vi "rsidr_core_global.vi"() -> ()   [LabVIEW 2015, in "Rohde&Schwarz CMXP NR FR2 Measurement.lvlib"] (continued)
"Access"=enum."Read Only", "Range Table"="", "Read Callback"="", "Write Callback"="", "Range Callback"="", "Check Callback"="", "Rngtable Callback"="", "Coerce Callback"="", "Supported Models"="", "Instrument Options"="", "Check Status Callback"="", "Flags"=0, "Help"="Returns equalizer spectrum flatness single value results (maximum within a range) for all measured list mode segments.\n\nAvailable Repeated Capabilities:\ninstance: i0, i1, i2, i3, i4, i5, i6, i7, i8, i9, i10, i11, i12, i13, i14, i15, i16, i17, i18, i19, i20, i21, i22, i23, i24, i25, i26, i27, i28, i29, i30, i31, i32\r\nRange: r1, r2\r\n\nRemote-control command(s):\nFETCh:NRMMw:MEAS<i>:MEValuation:LIST:ESFLatness:MAXR<no>:CURRent?"}, {"Level"=5, "Class Only"=FALSE, "Identifier"="RSCMXPNRFR2M_ATTR_FETCH_MULTI_EVAL_MEASUREMENT_LIST_ESF_MAXR_EXTREME_RESULTS", "Descriptive Name"="Fetch Multi Eval Measurement List ES Flatness MaxR Extreme Results", "Data Type"=enum."RawString", "Command"="FETC:NRMM:MEAS{instance}:MEV:LIST:ESFL:MAXR{Range}:EXTR?", "Access"=enum."Read Only", "Range Table"="", "Read Callback"="", "Write Callback"="", "Range Callback"="", "Check Callback"="", "Rngtable Callback"="", "Coerce Callback"="", "Supported Models"="", "Instrument Options"="", "Check Status Callback"="", "Flags"=0, "Help"="Returns equalizer spectrum flatness single value results (maximum within a range) for all measured list mode segments.\n\nAvailable Repeated Capabilities:\ninstance: i0, i1, i2, i3, i4, i5, i6, i7, i8, i9, i10, i11, i12, i13, i14, i15, i16, i17, i18, i19, i20, i21, i22, i23, i24, i25, i26, i27, i28, i29, i30, i31, i32\r\nRange: r1, r2\r\n\nRemote-control command(s):\nFETCh:NRMMw:MEAS<i>:MEValuation:LIST:ESFLatness:MAXR<no>:EXTReme?"}, {"Level"=5, "Class Only"=FALSE, "Identifier"="RSCMXPNRFR2M_ATTR_FETCH_MULTI_EVAL_MEASUREMENT_LIST_ESF_MAXR_STANDARD_DEVIATION_RESULTS", "Descriptive Name"="Fetch Multi Eval Measurement List ES Flatness MaxR Standard Deviation Results", "Data Type"=enum."RawString", "Command"="FETC:NRMM:MEAS{instance}:MEV:LIST:ESFL:MAXR{Range}:SDEV?", "Access"=enum."Read Only", "Range Table"="", "Read Callback"="", "Write Callback"="", "Range Callback"="", "Check Callback"="", "Rngtable Callback"="", "Coerce Callback"="", "Supported Models"="", "Instrument Options"="", "Check Status Callback"="", "Flags"=0, "Help"="Returns equalizer spectrum flatness single value results (maximum within a range) for all measured list mode segments.\n\nAvailable Repeated Capabilities:\ninstance: i0, i1, i2, i3, i4, i5, i6, i7, i8, i9, i10, i11, i12, i13, i14, i15, i16, i17, i18, i19, i20, i21, i22, i23, i24, i25, i26, i27, i28, i29, i30, i31, i32\r\nRange: r1, r2\r\n\nRemote-control command(s):\nFETCh:NRMMw:MEAS<i>:MEValuation:LIST:ESFLatness:MAXR<no>:SDEViation?"}, {"Level"=5, "Class Only"=FALSE, "Identifier"="RSCMXPNRFR2M_ATTR_QUERY_MULTI_EVAL_MEASUREMENT_LIST_ESF_MAXR_AVERAGE_LIMIT_CHECK_RESULTS", "Descriptive Name"="Query Multi Eval Measurement List ES Flatness MaxR Average Limit Check Results", "Data Type"=enum."RawString", "Command"="CALC:NRMM:MEAS{instance}:MEV:LIST:ESFL:MAXR{Range}:AVER?", "Access"=enum."Read Only", "Range Table"="", "Read Callback"="", "Write Callback"="", "Range Callback"="", "Check Callback"="", "Rngtable Callback"="", "Coerce Callback"="", "Supported Models"="", "Instrument Options"="", "Check Status Callback"="", "Flags"=0, "Help"="Returns the limit check results for equalizer spectrum flatness single value results (maximum within a range) for all measured list mode segments.\n\nAvailable Repeated Capabilities:\ninstance: i0, i1, i2, i3, i4, i5, i6, i7, i8, i9, i10, i11, i12, i13, i14, i15, i16, i17, i18, i19, i20, i21, i22, i23, i24, i25, i26, i27, i28, i29, i30, i31, i32\r\nRange: r1, r2\r\n\nRemote-control command(s):\nCALCulate:NRMMw:MEAS<i>:MEValuation:LIST:ESFLatness:MAXR<no>:AVERage?"}, {"Level"=5, "Class Only"=FALSE, "Identifier"="RSCMXPNRFR2M_ATTR_QUERY_MULTI_EVAL_MEASUREMENT_LIST_ESF_MAXR_CURRENT_LIMIT_CHECK_RESULTS", "Descriptive Name"="Query Multi Eval Measurement List ES Flatness MaxR Current Limit Check Results", "Data Type"=enum."RawString", "Command"="CALC:NRMM:MEAS{instance}:MEV:LIST:ESFL:MAXR{Range}:CURR?", "Access"=enum."Read Only", "Range Table"="", "Read Callback"="", "Write Callback"="", "Range Callback"="", "Check Callback"="", "Rngtable Callback"="", "Coerce Callback"="", "Supported Models"="", "Instrument Options"="", "Check Status Callback"="", "Flags"=0, "Help"="Returns the limit check results for equalizer spectrum flatness single value results (maximum within a range) for all measured list mode segments.\n\nAvailable Repeated Capabilities:\ninstance: i0, i1, i2, i3, i4, i5, i6, i7, i8, i9, i10, i11, i12, i13, i14, i15, i16, i17, i18, i19, i20, i21, i22, i23, i24, i25, i26, i27, i28, i29, i30, i31, i32\r\nRange: r1, r2\r\n\nRemote-control command(s):\nCALCulate:NRMMw:MEAS<i>:MEValuation:LIST:ESFLatness:MAXR<no>:CURRent?"}, {"Level"=5, "Class Only"=FALSE, "Identifier"="RSCMXPNRFR2M_ATTR_QUERY_MULTI_EVAL_MEASUREMENT_LIST_ESF_MAXR_EXTREME_LIMIT_CHECK_RESULTS", "Descriptive Name"="Query Multi Eval Measurement List ES Flatness MaxR Extreme Limit Check Results", "Data Type"=enum."RawString", "Command"="CALC:NRMM:MEAS{instance}:MEV:LIST:ESFL:MAXR{Range}:EXTR?", "Access"=enum."Read Only", "Range Table"="", "Read Callback"="", "Write Callback"="", "Range Callback"="", "Check Callback"="", "Rngtable Callback"="", "Coerce Callback"="", "Supported Models"="", "Instrument Options"="", "Check Status Callback"="", "Flags"=0, "Help"="Returns the limit check results for equalizer spectrum flatness single value results (maximum within a range) for all measured list mode segments.\n\nAvailable Repeated Capabilities:\ninstance: i0, i1, i2, i3, i4, i5, i6, i7, i8, i9, i10, i11, i12, i13, i14, i15, i16, i17, i18, i19, i20, i21, i22, i23, i24, i25, i26, i27, i28, i29, i30, i31, i32\r\nRange: r1, r2\r\n\nRemote-control command(s):\nCALCulate:NRMMw:MEAS<i>:MEValuation:LIST:ESFLatness:MAXR<no>:EXTReme?"}, {"Level"=5, "Class Only"=FALSE, "Identifier"="RSCMXPNRFR2M_ATTR_FETCH_MULTI_EVAL_MEASUREMENT_LIST_ESF_MINR_AVERAGE_RESULTS", "Descriptive Name"="Fetch Multi Eval Measurement List ES Flatness MinR Average Results", "Data Type"=enum."RawString", "Command"="FETC:NRMM:MEAS{instance}:MEV:LIST:ESFL:MINR{Range}:AVER?", "Access"=enum."Read Only", "Range Table"="", "Read Callback"="", "Write Callback"="", "Range Callback"="", "Check Callback"="", "Rngtable Callback"="", "Coerce Callback"="", "Supported Models"="", "Instrument Options"="", "Check Status Callback"="", "Flags"=0, "Help"="Returns equalizer spectrum flatness single value results (minimum within a range) for all measured list mode segments.\n\nAvailable Repeated Capabilities:\ninstance: i0, i1, i2, i3, i4, i5, i6, i7, i8, i9, i10, i11, i12, i13, i14, i15, i16, i17, i18, i19, i20, i21, i22, i23, i24, i25, i26, i27, i28, i29, i30, i31, i32\r\nRange: r1, r2\r\n\nRemote-control command(s):\nFETCh:NRMMw:MEAS<i>:MEValuation:LIST:ESFLatness:MINR<no>:AVERage?"}, {"Level"=5, "Class Only"=FALSE, "Identifier"="RSCMXPNRFR2M_ATTR_FETCH_MULTI_EVAL_MEASUREMENT_LIST_ESF_MINR_CURRENT_RESULTS", "Descriptive Name"="Fetch Multi Eval Measurement List ES Flatness MinR Current Results", "Data Type"=enum."RawString", "Command"="FETC:NRMM:MEAS{instance}:MEV:LIST:ESFL:MINR{Range}:CURR?", "Access"=enum."Read Only", "Range Table"="", "Read Callback"="", "Write Callback"="", "Range Callback"="", "Check Callback"="", "Rngtable Callback"="", "Coerce Callback"="", "Supported Models"="", "Instrument Options"="", "Check Status Callback"="", "Flags"=0, "Help"="Returns equalizer spectrum flatness single value results (minimum within a range) for all measured list mode segments.\n\nAvailable Repeated Capabilities:\ninstance: i0, i1, i2, i3, i4, i5, i6, i7, i8, i9, i10, i11, i12, i13, i14, i15, i16, i17, i18, i19, i20, i21, i22, i23, i24, i25, i26, i27, i28, i29, i30, i31, i32\r\nRange: r1, r2\r\n\nRemote-control command(s):\nFETCh:NRMMw:MEAS<i>:MEValuation:LIST:ESFLatness:MINR<no>:CURRent?"}, {"Level"=5, "Class Only"=FALSE, "Identifier"="RSCMXPNRFR2M_ATTR_FETCH_MULTI_EVAL_MEASUREMENT_LIST_ESF_MINR_EXTREME_RESULTS", "Descriptive Name"="Fetch Multi Eval Measurement List ES Flatness MinR Extreme Results", "Data Type"=enum."RawString", "Command"="FETC:NRMM:MEAS{instance}:MEV:LIST:ESFL:MINR{Range}:EXTR?", "Access"=enum."Read Only", "Range Table"="", "Read Callback"="", "Write Callback"="", "Range Callback"="", "Check Callback"="", "Rngtable Callback"="", "Coerce Callback"="", "Supported Models"="", "Instrument Options"="", "Check Status Callback"="", "Flags"=0, "Help"="Returns equalizer spectrum flatness single value results (minimum within a range) for all measured list mode segments.\n\nAvailable Repeated Capabilities:\ninstance: i0, i1, i2, i3, i4, i5, i6, i7, i8, i9, i10, i11, i12, i13, i14, i15, i16, i17, i18, i19, i20, i21, i22, i23, i24, i25, i26, i27, i28, i29, i30, i31, i32\r\nRange: r1, r2\r\n\nRemote-control command(s):\nFETCh:NRMMw:MEAS<i>:MEValuation:LIST:ESFLatness:MINR<no>:EXTReme?"}, {"Level"=5, "Class Only"=FALSE, "Identifier"="RSCMXPNRFR2M_ATTR_FETCH_MULTI_EVAL_MEASUREMENT_LIST_ESF_MINR_STANDARD_DEVIATION_RESULTS", "Descriptive Name"="Fetch Multi Eval Measurement List ES Flatness MinR Standard Deviation Results", "Data Type"=enum."RawString", "Command"="FETC:NRMM:MEAS{instance}:MEV:LIST:ESFL:MINR{Range}:SDEV?", "Access"=enum."Read Only", "Range Table"="", "Read Callback"="", "Write Callback"="", "Range Callback"="", "Check Callback"="", "Rngtable Callback"="", "Coerce Callback"="", "Supported Models"="", "Instrument Options"="", "Check Status Callback"="", "Flags"=0, "Help"="Returns equalizer spectrum flatness single value results (minimum within a range) for all measured list mode segments.\n\nAvailable Repeated Capabilities:\ninstance: i0, i1, i2, i3, i4, i5, i6, i7, i8, i9, i10, i11, i12, i13, i14, i15, i16, i17, i18, i19, i20, i21, i22, i23, i24, i25, i26, i27, i28, i29, i30, i31, i32\r\nRange: r1, r2\r\n\nRemote-control command(s):\nFETCh:NRMMw:MEAS<i>:MEValuation:LIST:ESFLatness:MINR<no>:SDEViation?"}, {"Level"=5, "Class Only"=FALSE, "Identifier"="RSCMXPNRFR2M_ATTR_QUERY_MULTI_EVAL_MEASUREMENT_LIST_ESF_MINR_AVERAGE_LIMIT_CHECK_RESULTS", "Descriptive Name"="Query Multi Eval Measurement List ES Flatness MinR Average Limit Check Results", "Data Type"=enum."RawString", "Command"="CALC:NRMM:MEAS{instance}:MEV:LIST:ESFL:MINR{Range}:AVER?", "Access"=enum."Read Only", "Range Table"="", "Read Callback"="", "Write Callback"="", "Range Callback"="", "Check Callback"="", "Rngtable Callback"="", "Coerce Callback"="", "Supported Models"="", "Instrument Options"="", "Check Status Callback"="", "Flags"=0, "Help"="Returns the limit check results for equalizer spectrum flatness single value results (minimum within a range) for all measured list mode segments.\n\nAvailable Repeated Capabilities:\ninstance: i0, i1, i2, i3, i4, i5, i6, i7, i8, i9, i10, i11, i12, i13, i14, i15, i16, i17, i18, i19, i20, i21, i22, i23, i24, i25, i26, i27, i28, i29, i30, i31, i32\r\nRange: r1, r2\r\n\nRemote-control command(s):\nCALCulate:NRMMw:MEAS<i>:MEValuation:LIST:ESFLatness:MINR<no>:AVERage?"}, {"Level"=5, "Class Only"=FALSE, "Identifier"="RSCMXPNRFR2M_ATTR_QUERY_MULTI_EVAL_MEASUREMENT_LIST_ESF_MINR_CURRENT_LIMIT_CHECK_RESULTS", "Descriptive Name"="Query Multi Eval Measurement List ES Flatness MinR Current Limit Check Results", "Data Type"=enum."RawString", "Command"="CALC:NRMM:MEAS{instance}:MEV:LIST:ESFL:MINR{Range}:CURR?", "Access"=enum."Read Only", "Range Table"="", "Read Callback"="", "Write Callback"="", "Range Callback"="", "Check Callback"="", "Rngtable Callback"="", "Coerce Callback"="", "Supported Models"="", "Instrument Options"="", "Check Status Callback"="", "Flags"=0, "Help"="Returns the limit check results for equalizer spectrum flatness single value results (minimum within a range) for all measured list mode segments.\n\nAvailable Repeated Capabilities:\ninstance: i0, i1, i2, i3, i4, i5, i6, i7, i8, i9, i10, i11, i12, i13, i14, i15, i16, i17, i18, i19, i20, i21, i22, i23, i24, i25, i26, i27, i28, i29, i30, i31, i32\r\nRange: r1, r2\r\n\nRemote-control command(s):\nCALCulate:NRMMw:MEAS<i>:MEValuation:LIST:ESFLatness:MINR<no>:CURRent?"}, {"Level"=5, "Class Only"=FALSE, "Identifier"="RSCMXPNRFR2M_ATTR_QUERY_MULTI_EVAL_MEASUREMENT_LIST_ESF_MINR_EXTREME_LIMIT_CHECK_RESULTS", "Descriptive Name"="Query Multi Eval Measurement List ES Flatness MinR Extreme Limit Check Results", "Data Type"=enum."RawString", "Command"="CALC:NRMM:MEAS{instance}:MEV:LIST:ESFL:MINR{Range}:EXTR?", "Access"=enum."Read Only", "Range Table"="", "Read Callback"="", "Write Callback"="", "Range Callback"="", "Check Callback"="", "Rngtable Callback"="", "Coerce Callback"="", "Supported Models"="", "Instrument Options"="", "Check Status Callback"="", "Flags"=0, "Help"="Returns the limit check results for equalizer spectrum flatness single value results (minimum within a range) for all measured list mode segments.\n\nAvailable Repeated Capabilities:\ninstance: i0, i1, i2, i3, i4, i5, i6, i7, i8, i9, i10, i11, i12, i13, i14, i15, i16, i17, i18, i19, i20, i21, i22, i23, i24, i25, i26, i27, i28, i29, i30, i31, i32\r\nRange: r1, r2\r\n\nRemote-control command(s):\nCALCulate:NRMMw:MEAS<i>:MEValuation:LIST:ESFLatness:MINR<no>:EXTReme?"}, {"Level"=5, "Class Only"=FALSE, "Identifier"="RSCMXPNRFR2M_ATTR_FETCH_MULTI_EVAL_MEASUREMENT_LIST_ESF_RIPPLE_AVERAGE_RESULTS", "Descriptive Name"="Fetch Multi Eval Measurement List ES Flatness Ripple Average Results", "Data Type"=enum."RawString", "Command"="FETC:NRMM:MEAS{instance}:MEV:LIST:ESFL:RIPP{Ripple}:AVER?", "Access"=enum."Read Only", "Range Table"="", "Read Callback"="", "Write Callback"="", "Range Callback"="", "Check Callback"="", "Rngtable Callback"="", "Coerce Callback"="", "Supported Models"="", "Instrument Options"="", "Check Status Callback"="", "Flags"=0, "Help"="Returns equalizer spectrum flatness single value results (ripple 1 or ripple 2) for all measured list mode segments.\n\nAvailable Repeated Capabilities:\ninstance: i0, i1, i2, i3, i4, i5, i6, i7, i8, i9, i10, i11, i12, i13, i14, i15, i16, i17, i18, i19, i20, i21, i22, i23, i24, i25, i26, i27, i28, i29, i30, i31, i32\r\nRipple: r1, r2\r\n\nRemote-control command(s):\nFETCh:NRMMw:MEAS<i>:MEValuation:LIST:ESFLatness:RIPPle<no>:AVERage?"}, {"Level"=5, "Class Only"=FALSE, "Identifier"="RSCMXPNRFR2M_ATTR_FETCH_MULTI_EVAL_MEASUREMENT_LIST_ESF_RIPPLE_CURRENT_RESULTS", "Descriptive Name"="Fetch Multi Eval Measurement List ES Flatness Ripple Current Results", "Data Type"=enum."RawString", "Command"="FETC:NRMM:MEAS{instance}:MEV:LIST:ESFL:RIPP{Ripple}:CURR?", "Access"=enum."Read Only", "Range Table"="", "Read Callback"="", "Write Callback"="", "Range Callback"="", "Check Callback"="", "Rngtable Callback"="", "Coerce Callback"="", "Supported Models"="", "Instrument Options"="", "Check Status Callback"="", "Flags"=0, "Help"="Returns equalizer spectrum flatness single value results (ripple 1 or ripple 2) for all measured list mode segments.\n\nAvailable Repeated Capabilities:\ninstance: i0, i1, i2, i3, i4, i5, i6, i7, i8, i9, i10, i11, i12, i13, i14, i15, i16, i17, i18, i19, i20, i21, i22, i23, i24, i25, i26, i27, i28, i29, i30, i31, i32\r\nRipple: r1, r2\r\n\nRemote-control command(s):\nFETCh:NRMMw:MEAS<i>:MEValuation:LIST:ESFLatness:RIPPle<no>:CURRent?"}, {"Level"=5, "Class Only"=FALSE, "Identifier"="RSCMXPNRFR2M_ATTR_FETCH_MULTI_EVAL_MEASUREMENT_LIST_ESF_RIPPLE_EXTREME_RESULTS", "Descriptive Name"="Fetch Multi Eval Measurement List ES Flatness Ripple Extreme Results", "Data Type"=enum."RawString", "Command"="FETC:NRMM:MEAS{instance}:MEV:LIST:ESFL:RIPP{Ripple}:EXTR?", "Access"=enum."Read Only", "Range Table"="", "Read Callback"="", "Write Callback"="", "Range Callback"="", "Check Callback"="", "Rngtable Callback"="", "Coerce Callback"="", "Supported Models"="", "Instrument Options"="", "Check Status Callback"="", "Flags"=0, "Help"="Returns equalizer spectrum flatness single value results (ripple 1 or ripple 2) for all measured list mode segments.\n\nAvailable Repeated Capabilities:\ninstance: i0, i1, i2, i3, i4, i5, i6, i7, i8, i9, i10, i11, i12, i13, i14, i15, i16, i17, i18, i19, i20, i21, i22, i23, i24, i25, i26, i27, i28, i29, i30, i31, i32\r\nRipple: r1, r2\r\n\nRemote-control command(s):\nFETCh:NRMMw:MEAS<i>:MEValuation:LIST:ESFLatness:RIPPle<no>:EXTReme?"}, {"Level"=5, "Class Only"=FALSE, "Identifier"="RSCMXPNRFR2M_ATTR_FETCH_MULTI_EVAL_MEASUREMENT_LIST_ESF_RIPPLE_STANDARD_DEVIATION_RESULTS", "Descriptive Name"="Fetch Multi Eval Measurement List ES Flatness Ripple Standard Deviation Results", "Data Type"=enum."RawString", "Command"="FETC:NRMM:MEAS{instance}:MEV:LIST:ESFL:RIPP{Ripple}:SDEV?", "Access"=enum."Read Only", "Range Table"="", "Read Callback"="", "Write Callback"="", "Range Callback"="", "Check Callback"="", "Rngtable Callback"="", "Coerce Callback"="", "Supported Models"="", "Instrument Options"="", "Check Status Callback"="", "Flags"=0, "Help"="Returns equalizer spectrum flatness single value results (ripple 1 or ripple 2) for all measured list mode segments.\n\nAvailable Repeated Capabilities:\ninstance: i0, i1, i2, i3, i4, i5, i6, i7, i8, i9, i10, i11, i12, i13, i14, i15, i16, i17, i18, i19, i20, i21, i22, i23, i24, i25, i26, i27, i28, i29, i30, i31, i32\r\nRipple: r1, r2\r\n\nRemote-control command(s):\nFETCh:NRMMw:MEAS<i>:MEValuation:LIST:ESFLatness:RIPPle<no>:SDEViation?"}, {"Level"=5, "Class Only"=FALSE, "Identifier"="RSCMXPNRFR2M_ATTR_QUERY_MULTI_EVAL_MEASUREMENT_LIST_ESF_RIPPLE_AVERAGE_LIMIT_CHECK_RESULTS", "Descriptive Name"="Query Multi Eval Measurement List ES Flatness Ripple Average Limit Check Results", "Data Type"=enum."RawString", "Command"="CALC:NRMM:MEAS{instance}:MEV:LIST:ESFL:RIPP{Ripple}:AVER?", "Access"=enum."Read Only", "Range Table"="", "Read Callback"="", "Write Callback"="", "Range Callback"="", "Check Callback"="", "Rngtable Callback"="", "Coerce Callback"="", "Supported Models"="", "Instrument Options"="", "Check Status Callback"="", "Flags"=0, "Help"="Returns the limit check results for equalizer spectrum flatness single value results (ripple 1 or ripple 2) for all measured list mode segments.\n\nAvailable Repeated Capabilities:\ninstance: i0, i1, i2, i3, i4, i5, i6, i7, i8, i9, i10, i11, i12, i13, i14, i15, i16, i17, i18, i19, i20, i21, i22, i23, i24, i25, i26, i27, i28, i29, i30, i31, i32\r\nRipple: r1, r2\r\n\nRemote-control command(s):\nCALCulate:NRMMw:MEAS<i>:MEValuation:LIST:ESFLatness:RIPPle<no>:AVERage?"}, {"Level"=5, "Class Only"=FALSE, "Identifier"="RSCMXPNRFR2M_ATTR_QUERY_MULTI_EVAL_MEASUREMENT_LIST_ESF_RIPPLE_CURRENT_LIMIT_CHECK_RESULTS", "Descriptive Name"="Query Multi Eval Measurement List ES Flatness Ripple Current Limit Check Results", "Data Type"=enum."RawString", "Command"="CALC:NRMM:MEAS{instance}:MEV:LIST:ESFL:RIPP{Ripple}:CURR?", "Access"=enum."Read Only", "Range Table"="", "Read Callback"="", "Write Callback"="", "Range Callback"="", "Check Callback"="", "Rngtable Callback"="", "Coerce Callback"="", "Supported Models"="", "Instrument Options"="", "Check Status Callback"="", "Flags"=0, "Help"="Returns the limit check results for equalizer spectrum flatness single value results (ripple 1 or ripple 2) for all measured list mode segments.\n\nAvailable Repeated Capabilities:\ninstance: i0, i1, i2, i3, i4, i5, i6, i7, i8, i9, i10, i11, i12, i13, i14, i15, i16, i17, i18, i19, i20, i21, i22, i23, i24, i25, i26, i27, i28, i29, i30, i31, i32\r\nRipple: r1, r2\r\n\nRemote-control command(s):\nCALCulate:NRMMw:MEAS<i>:MEValuation:LIST:ESFLatness:RIPPle<no>:CURRent?"}, {"Level"=5, "Class Only"=FALSE, "Identifier"="RSCMXPNRFR2M_ATTR_QUERY_MULTI_EVAL_MEASUREMENT_LIST_ESF_RIPPLE_EXTREME_LIMIT_CHECK_RESULTS", "Descriptive Name"="Query Multi Eval Measurement List ES Flatness Ripple Extreme Limit Check Results", "Data Type"=enum."RawString", "Command"="CALC:NRMM:MEAS{instance}:MEV:LIST:ESFL:RIPP{Ripple}:EXTR?", "Access"=enum."Read Only", "Range Table"="", "Read Callback"="", "Write Callback"="", "Range Callback"="", "Check Callback"="", "Rngtable Callback"="", "Coerce Callback"="", "Supported Models"="", "Instrument Options"="", "Check Status Callback"="", "Flags"=0, "Help"="Returns the limit check results for equalizer spectrum flatness single value results (ripple 1 or ripple 2) for all measured list mode segments.\n\nAvailable Repeated Capabilities:\ninstance: i0, i1, i2, i3, i4, i5, i6, i7, i8, i9, i10, i11, i12, i13, i14, i15, i16, i17, i18, i19, i20, i21, i22, i23, i24, i25, i26, i27, i28, i29, i30, i31, i32\r\nRipple: r1, r2\r\n\nRemote-control command(s):\nCALCulate:NRMMw:MEAS<i>:MEValuation:LIST:ESFLatness:RIPPle<no>:EXTReme?"}, {"Level"=5, "Class Only"=FALSE, "Identifier"="RSCMXPNRFR2M_ATTR_FETCH_MULTI_EVAL_MEASUREMENT_LIST_ESF_SCINDEX_MAXIMUM_CURRENT_RESULTS", "Descriptive Name"="Fetch Multi Eval Measurement List ES Flatness Subcarrier Index Maximum Current Results", "Data Type"=enum."RawString", "Command"="FETC:NRMM:MEAS{instance}:MEV:LIST:ESFL:SCIN:MAX{Range}:CURR?", "Access"=enum."Read Only", "Range Table"="", "Read Callback"="", "Write Callback"="", "Range Callback"="", "Check Callback"="", "Rngtable Callback"="", "Coerce Callback"="", "Supported Models"="", "Instrument Options"="", "Check Status Callback"="", "Flags"=0, "Help"="Returns subcarrier indices of the equalizer spectrum flatness measurement for all measured list mode segments.\n\nAvailable Repeated Capabilities:\ninstance: i0, i1, i2, i3, i4, i5, i6, i7, i8, i9, i10, i11, i12, i13, i14, i15, i16, i17, i18, i19, i20, i21, i22, i23, i24, i25, i26, i27, i28, i29, i30, i31, i32\r\nRange: r1, r2\r\n\nRemote-control command(s):\nFETCh:NRMMw:MEAS<i>:MEValuation:LIST:ESFLatness:SCINdex:MAXimum<no>:CURRent?"}, {"Level"=5, "Class Only"=FALSE, "Identifier"="RSCMXPNRFR2M_ATTR_FETCH_MULTI_EVAL_MEASUREMENT_LIST_ESF_SCINDEX_MINIMUM_CURRENT_RESULTS", "Descriptive Name"="Fetch Multi Eval Measurement List ES Flatness Subcarrier Index Minimum Current Results", "Data Type"=enum."RawString", "Command"="FETC:NRMM:MEAS{instance}:MEV:LIST:ESFL:SCIN:MIN{Range}:CURR?", "Access"=enum."Read Only", "Range Table"="", "Read Callback"="", "Write Callback"="", "Range Callback"="", "Check Callback"="", "Rngtable Callback"="", "Coerce Callback"="", "Supported Models"="", "Instrument Options"="", "Check Status Callback"="", "Flags"=0, "Help"="Returns subcarrier indices of the equalizer spectrum flatness measurement for all measured list mode segments.\n\nAvailable Repeated Capabilities:\ninstance: i0, i1, i2, i3, i4, i5, i6, i7, i8, i9, i10, i11, i12, i13, i14, i15, i16, i17, i18, i19, i20, i21, i22, i23, i24, i25, i26, i27, i28, i29, i30, i31, i32\r\nRange: r1, r2\r\n\nRemote-control command(s):\nFETCh:NRMMw:MEAS<i>:MEValuation:LIST:ESFLatness:SCINdex:MINimum<no>:CURRent?"}, {"Level"=4, "Class Only"=TRUE, "Identifier"="", "Descriptive Name"="Error Vector Magnitude", "Data Type"=enum."ViInt32", "Command"="", "Access"=enum."Read Only", "Range Table"="", "Read Callback"="", "Write Callback"="", "Range Callback"="", "Check Callback"="", "Rngtable Callback"="", "Coerce Callback"="", "Supported Models"="", "Instrument Options"="", "Check Status Callback"="", "Flags"=0, "Help"="The following attributes return error vector magnitude values for low and high EVM window position, for all measured list mode segments."}, {"Level"=5, "Class Only"=FALSE, "Identifier"="RSCMXPNRFR2M_ATTR_FETCH_MULTI_EVAL_MEASUREMENT_LIST_EVM_DMRS_HIGH_AVERAGE_RESULTS", "Descriptive Name"="Fetch Multi Eval Measurement List EVM DMRS High Average Results", "Data Type"=enum."RawString", "Command"="FETC:NRMM:MEAS{instance}:MEV:LIST:MOD:EVM:DMRS:HIGH:AVER?", "Access"=enum."Read Only", "Range Table"="", "Read Callback"="", "Write Callback"="", "Range Callback"="", "Check Callback"="", "Rngtable Callback"="", "Coerce Callback"="", "Supported Models"="", "Instrument Options"="", "Check Status Callback"="", "Flags"=0, "Help"="Returns error vector magnitude DMRS values for low and high EVM window position, for all measured list mode segments.\n\nAvailable Repeated Capabilities:\ninstance: i0, i1, i2, i3, i4, i5, i6, i7, i8, i9, i10, i11, i12, i13, i14, i15, i16, i17, i18, i19, i20, i21, i22, i23, i24, i25, i26, i27, i28, i29, i30, i31, i32\r\n\nRemote-control command(s):\nFETCh:NRMMw:MEAS<i>:MEValuation:LIST:MODulation:EVM:DMRS:HIGH:AVERage?"}, {"Level"=5, "Class Only"=FALSE, "Identifier"="RSCMXPNRFR2M_ATTR_FETCH_MULTI_EVAL_MEASUREMENT_LIST_EVM_DMRS_HIGH_CURRENT_RESULTS", "Descriptive Name"="Fetch Multi Eval Measurement List EVM DMRS High Current Results", "Data Type"=enum."RawString", "Command"="FETC:NRMM:MEAS{instance}:MEV:LIST:MOD:EVM:DMRS:HIGH:CURR?", "Access"=enum."Read Only", "Range Table"="", "Read Callback"="", "Write Callback"="", "Range Callback"="", "Check Callback"="", "Rngtable Callback"="", "Coerce Callback"="", "Supported Models"="", "Instrument Options"="", "Check Status Callback"="", "Flags"=0, "Help"="Returns error vector magnitude DMRS values for low and high EVM window position, for all measured list mode segments.\n\nAvailable Repeated Capabilities:\ninstance: i0, i1, i2, i3, i4, i5, i6, i7, i8, i9, i10, i11, i12, i13, i14, i15, i16, i17, i18, i19, i20, i21, i22, i23, i24, i25, i26, i27, i28, i29, i30, i31, i32\r\n\nRemote-control command(s):\nFETCh:NRMMw:MEAS<i>:MEValuation:LIST:MODulation:EVM:DMRS:HIGH:CURRent?"}, {"Level"=5, "Class Only"=FALSE, "Identifier"="RSCMXPNRFR2M_ATTR_FETCH_MULTI_EVAL_MEASUREMENT_LIST_EVM_DMRS_HIGH_EXTREME_RESULTS", "Descriptive Name"="Fetch Multi Eval Measurement List EVM DMRS High Extreme Results", "Data Type"=enum."RawString", "Command"="FETC:NRMM:MEAS{instance}:MEV:LIST:MOD:EVM:DMRS:HIGH:EXTR?", "Access"=enum."Read Only", "Range Table"="", "Read Callback"="", "Write Callback"="", "Range Callback"="", "Check Callback"="", "Rngtable Callback"="", "Coerce Callback"="", "Supported Models"="", "Instrument Options"="", "Check Status Callback"="", "Flags"=0, "Help"="Returns error vector magnitude DMRS values for low and high EVM window position, for all measured list mode segments.\n\nAvailable Repeated Capabilities:\ninstance: i0, i1, i2, i3, i4, i5, i6, i7, i8, i9, i10, i11, i12, i13, i14, i15, i16, i17, i18, i19, i20, i21, i22, i23, i24, i25, i26, i27, i28, i29, i30, i31, i32\r\n\nRemote-control command(s):\nFETCh:NRMMw:MEAS<i>:MEValuation:LIST:MODulation:EVM:DMRS:HIGH:EXTReme?"}, {"Level"=5, "Class Only"=FALSE, "Identifier"="RSCMXPNRFR2M_ATTR_FETCH_MULTI_EVAL_MEASUREMENT_LIST_EVM_DMRS_HIGH_STANDARD_DEVIATION_RESULTS", "Descriptive Name"="Fetch Multi Eval Measurement List EVM DMRS High Standard Deviation Results", "Data Type"=enum."RawString", "Command"="FETC:NRMM:MEAS{instance}:MEV:LIST:MOD:EVM:DMRS:HIGH:SDEV?", "Access"=enum."Read Only", "Range Table"="", "Read Callback"="", "Write Callback"="", "Range Callback"="", "Check Callback"="", "Rngtable Callback"="", "Coerce Callback"="", "Supported Models"="", "Instrument Options"="", "Check Status Callback"="", "Flags"=0, "Help"="Returns error vector magnitude DMRS values for low and high EVM window position, for all measured list mode segments.\n\nAvailable Repeated Capabilities:\ninstance: i0, i1, i2, i3, i4, i5, i6, i7, i8, i9, i10, i11, i12, i13, i14, i15, i16, i17, i18, i19, i20, i21, i22, i23, i24, i25, i26, i27, i28, i29, i30, i31, i32\r\n\nRemote-control command(s):\nFETCh:NRMMw:MEAS<i>:MEValuation:LIST:MODulation:EVM:DMRS:HIGH:SDEViation?"}, {"Level"=5, "Class Only"=FALSE, "Identifier"="RSCMXPNRFR2M_ATTR_FETCH_MULTI_EVAL_MEASUREMENT_LIST_EVM_DMRS_LOW_AVERAGE_RESULTS", "Descriptive Name"="Fetch Multi Eval Measurement List EVM DMRS Low Average Results", "Data Type"=enum."RawString", "Command"="FETC:NRMM:MEAS{instance}:MEV:LIST:MOD:EVM:DMRS:LOW:AVER?", "Access"=enum."Read Only", "Range Table"="", "Read Callback"="", "Write Callback"="", "Range Callback"="", "Check Callback"="", "Rngtable Callback"="", "Coerce Callback"="", "Supported Models"="", "Instrument Options"="", "Check Status Callback"="", "Flags"=0, "Help"="Returns error vector magnitude DMRS values for low and high EVM window position, for all measured list mode segments.\n\nAvailable Repeated Capabilities:\ninstance: i0, i1, i2, i3, i4, i5, i6, i7, i8, i9, i10, i11, i12, i13, i14, i15, i16, i17, i18, i19, i20, i21, i22, i23, i24, i25, i26, i27, i28, i29, i30, i31, i32\r\n\nRemote-control command(s):\nFETCh:NRMMw:MEAS<i>:MEValuation:LIST:MODulation:EVM:DMRS:LOW:AVERage?"}, {"Level"=5, "Class Only"=FALSE, "Identifier"="RSCMXPNRFR2M_ATTR_FETCH_MULTI_EVAL_MEASUREMENT_LIST_EVM_DMRS_LOW_CURRENT_RESULTS", "Descriptive Name"="Fetch Multi Eval Measurement List EVM DMRS Low Current Results", "Data Type"=enum."RawString", "Command"="FETC:NRMM:MEAS{instance}:MEV:LIST:MOD:EVM:DMRS:LOW:CURR?", "Access"=enum."Read Only", "Range Table"="", "Read Callback"="", "Write Callback"="", "Range Callback"="", "Check Callback"="", "Rngtable Callback"="", "Coerce Callback"="", "Supported Models"="", "Instrument Options"="", "Check Status Callback"="", "Flags"=0, "Help"="Returns error vector magnitude DMRS values for low and high EVM window position, for all measured list mode segments.\n\nAvailable Repeated Capabilities:\ninstance: i0, i1, i2, i3, i4, i5, i6, i7, i8, i9, i10, i11, i12, i13, i14, i15, i16, i17, i18, i19, i20, i21, i22, i23, i24, i25, i26, i27, i28, i29, i30, i31, i32\r\n\nRemote-control command(s):\nFETCh:NRMMw:MEAS<i>:MEValuation:LIST:MODulation:EVM:DMRS:LOW:CURRent?"}, {"Level"=5, "Class Only"=FALSE, "Identifier"="RSCMXPNRFR2M_ATTR_FETCH_MULTI_EVAL_MEASUREMENT_LIST_EVM_DMRS_LOW_EXTREME_RESULTS", "Descriptive Name"="Fetch Multi Eval Measurement List EVM DMRS Low Extreme Results", "Data Type"=enum."RawString", "Command"="FETC:NRMM:MEAS{instance}:MEV:LIST:MOD:EVM:DMRS:LOW:EXTR?", "Access"=enum."Read Only", "Range Table"="", "Read Callback"="", "Write Callback"="", "Range Callback"="", "Check Callback"="", "Rngtable Callback"="", "Coerce Callback"="", "Supported Models"="", "Instrument Options"="", "Check Status Callback"="", "Flags"=0, "Help"="Returns error vector magnitude DMRS values for low and high EVM window position, for all measured list mode segments.\n\nAvailable Repeated Capabilities:\ninstance: i0, i1, i2, i3, i4, i5, i6, i7, i8, i9, i10, i11, i12, i13, i14, i15, i16, i17, i18, i19, i20, i21, i22, i23, i24, i25, i26, i27, i28, i29, i30, i31, i32\r\n\nRemote-control command(s):\nFETCh:NRMMw:MEAS<i>:MEValuation:LIST:MODulation:EVM:DMRS:LOW:EXTReme?"}, {"Level"=5, "Class Only"=FALSE, "Identifier"="RSCMXPNRFR2M_ATTR_FETCH_MULTI_EVAL_MEASUREMENT_LIST_EVM_DMRS_LOW_STANDARD_DEVIATION_RESULTS", "Descriptive Name"="Fetch Multi Eval Measurement List EVM DMRS Low Standard Deviation Results", "Data Type"=enum."RawString", "Command"="FETC:NRMM:MEAS{instance}:MEV:LIST:MOD:EVM:DMRS:LOW:SDEV?", "Access"=enum."Read Only", "Range Table"="", "Read Callback"="", "Write Callback"="", "Range Callback"="", "Check Callback"="", "Rngtable Callback"="", "Coerce Callback"="", "Supported Models"="", "Instrument Options"="", "Check Status Callback"="", "Flags"=0, "Help"="Returns error vector magnitude DMRS values for low and high EVM window position, for all measured list mode segments.\n\nAvailable Repeated Capabilities:\ninstance: i0, i1, i2, i3, i4, i5, i6, i7, i8, i9, i10, i11, i12, i13, i14, i15, i16, i17, i18, i19, i20, i21, i22, i23, i24, i25, i26, i27, i28, i29, i30, i31, i32\r\n\nRemote-control command(s):\nFETCh:NRMMw:MEAS<i>:MEValuation:LIST:MODulation:EVM:DMRS:LOW:SDEViation?"}, {"Level"=5, "Class Only"=FALSE, "Identifier"="RSCMXPNRFR2M_ATTR_QUERY_MULTI_EVAL_MEASUREMENT_LIST_EVM_DMRS_HIGH_AVERAGE_LIMIT_CHECK_RESULTS", "Descriptive Name"="Query Multi Eval Measurement List EVM DMRS High Average Limit Check Results", "Data Type"=enum."RawString", "Command"="CALC:NRMM:MEAS{instance}:MEV:LIST:MOD:EVM:DMRS:HIGH:AVER?", "Access"=enum."Read Only", "Range Table"="", "Read Callback"="", "Write Callback"="", "Range Callback"="", "Check Callback"="", "Rngtable Callback"="", "Coerce Callback"="", "Supported Models"="", "Instrument Options"="", "Check Status Callback"="", "Flags"=0, "Help"="Returns the limit check results for error vector magnitude DMRS values for low and high EVM window position, for all measured list mode segments.\n\nAvailable Repeated Capabilities:\ninstance: i0, i1, i2, i3, i4, i5, i6, i7, i8, i9, i10, i11, i12, i13, i14, i15, i16, i17, i18, i19, i20, i21, i22, i23, i24, i25, i26, i27, i28, i29, i30, i31, i32\r\n\nRemote-control command(s):\nCALCulate:NRMMw:MEAS<i>:MEValuation:LIST:MODulation:EVM:DMRS:HIGH:AVERage?"}, {"Level"=5, "Class Only"=FALSE, "Identifier"="RSCMXPNRFR2M_ATTR_QUERY_MULTI_EVAL_MEASUREMENT_LIST_EVM_DMRS_HIGH_CURRENT_LIMIT_CHECK_RESULTS", "Descriptive Name"="Query Multi Eval Measurement List EVM DMRS High Current Limit Check Results", "Data Type"=enum."RawString", "Command"="CALC:NRMM:MEAS{instance}:MEV:LIST:MOD:EVM:DMRS:HIGH:CURR?", "Access"=enum."Read Only", "Range Table"="", "Read Callback"="", "Write Callback"="", "Range Callback"="", "Check Callback"="", "Rngtable Callback"="", "Coerce Callback"="", "Supported Models"="", "Instrument Options"="", "Check Status Callback"="", "Flags"=0, "Help"="Returns the limit check results for error vector magnitude DMRS values for low and high EVM window position, for all measured list mode segments.\n\nAvailable Repeated Capabilities:\ninstance: i0, i1, i2, i3, i4, i5, i6, i7, i8, i9, i10, i11, i12, i13, i14, i15, i16, i17, i18, i19, i20, i21, i22, i23, i24, i25, i26, i27, i28, i29, i30, i31, i32\r\n\nRemote-control command(s):\nCALCulate:NRMMw:MEAS<i>:MEValuation:LIST:MODulation:EVM:DMRS:HIGH:CURRent?"}, {"Level"=5, "Class Only"=FALSE, "Identifier"="RSCMXPNRFR2M_ATTR_QUERY_MULTI_EVAL_MEASUREMENT_LIST_EVM_DMRS_HIGH_EXTREME_LIMIT_CHECK_RESULTS", "Descriptive Name"="Query Multi Eval Measurement List EVM DMRS High Extreme Limit Check Results", "Data Type"=enum."RawString", "Command"="CALC:NRMM:MEAS{instance}:MEV:LIST:MOD:EVM:DMRS:HIGH:EXTR?", "Access"=enum."Read Only", "Range Table"="", "Read Callback"="", "Write Callback"="", "Range Callback"="", "Check Callback"="", "Rngtable Callback"="", "Coerce Callback"="", "Supported Models"="", "Instrument Options"="", "Check Status Callback"="", "Flags"=0, "Help"="Returns the limit check results for error vector magnitude DMRS values for low and high EVM window position, for all measured list mode segments.\n\nAvailable Repeated Capabilities:\ninstance: i0, i1, i2, i3, i4, i5, i6, i7, i8, i9, i10, i11, i12, i13, i14, i15, i16, i17, i18, i19, i20, i21, i22, i23, i24, i25, i26, i27, i28, i29, i30, i31, i32\r\n\nRemote-control command(s):\nCALCulate:NRMMw:MEAS<i>:MEValuation:LIST:MODulation:EVM:DMRS:HIGH:EXTReme?"}, {"Level"=5, "Class Only"=FALSE, "Identifier"="RSCMXPNRFR2M_ATTR_QUERY_MULTI_EVAL_MEASUREMENT_LIST_EVM_DMRS_LOW_AVERAGE_LIMIT_CHECK_RESULTS", "Descriptive Name"="Query Multi Eval Measurement List EVM DMRS Low Average Limit Check Results", "Data Type"=enum."RawString", "Command"="CALC:NRMM:MEAS{instance}:MEV:LIST:MOD:EVM:DMRS:LOW:AVER?", "Access"=enum."Read Only", "Range Table"="", "Read Callback"="", "Write Callback"="", "Range Callback"="", "Check Callback"="", "Rngtable Callback"="", "Coerce Callback"="", "Supported Models"="", "Instrument Options"="", "Check Status Callback"="", "Flags"=0, "Help"="Returns the limit check results for error vector magnitude DMRS values for low and high EVM window position, for all measured list mode segments.\n\nAvailable Repeated Capabilities:\ninstance: i0, i1, i2, i3, i4, i5, i6, i7, i8, i9, i10, i11, i12, i13, i14, i15, i16, i17, i18, i19, i20, i21, i22, i23, i24, i25, i26, i27, i28, i29, i30, i31, i32\r\n\nRemote-control command(s):\nCALCulate:NRMMw:MEAS<i>:MEValuation:LIST:MODulation:EVM:DMRS:LOW:AVERage?"}, {"Level"=5, "Class Only"=FALSE, "Identifier"="RSCMXPNRFR2M_ATTR_QUERY_MULTI_EVAL_MEASUREMENT_LIST_EVM_DMRS_LOW_CURRENT_LIMIT_CHECK_RESULTS", "Descriptive Name"="Query Multi Eval Measurement List EVM DMRS Low Current Limit Check Results", "Data Type"=enum."RawString", "Command"="CALC:NRMM:MEAS{instance}:MEV:LIST:MOD:EVM:DMRS:LOW:CURR?", "Access"=enum."Read Only", "Range Table"="", "Read Callback"="", "Write Callback"="", "Range Callback"="", "Check Callback"="", "Rngtable Callback"="", "Coerce Callback"="", "Supported Models"="", "Instrument Options"="", "Check Status Callback"="", "Flags"=0, "Help"="Returns the limit check results for error vector magnitude DMRS values for low and high EVM window position, for all measured list mode segments.\n\nAvailable Repeated Capabilities:\ninstance: i0, i1, i2, i3, i4, i5, i6, i7, i8, i9, i10, i11, i12, i13, i14, i15, i16, i17, i18, i19, i20, i21, i22, i23, i24, i25, i26, i27, i28, i29, i30, i31, i32\r\n\nRemote-control command(s):\nCALCulate:NRMMw:MEAS<i>:MEValuation:LIST:MODulation:EVM:DMRS:LOW:CURRent?"}, {"Level"=5, "Class Only"=FALSE, "Identifier"="RSCMXPNRFR2M_ATTR_QUERY_MULTI_EVAL_MEASUREMENT_LIST_EVM_DMRS_LOW_EXTREME_LIMIT_CHECK_RESULTS", "Descriptive Name"="Query Multi Eval Measurement List EVM DMRS Low Extreme Limit Check Results", "Data Type"=enum."RawString", "Command"="CALC:NRMM:MEAS{instance}:MEV:LIST:MOD:EVM:DMRS:LOW:EXTR?", "Access"=enum."Read Only", "Range Table"="", "Read Callback"="", "Write Callback"="", "Range Callback"="", "Check Callback"="", "Rngtable Callback"="", "Coerce Callback"="", "Supported Models"="", "Instrument Options"="", "Check Status Callback"="", "Flags"=0, "Help"="Returns the limit check results for error vector magnitude DMRS values for low and high EVM window position, for all measured list mode segments.\n\nAvailable Repeated Capabilities:\ninstance: i0, i1, i2, i3, i4, i5, i6, i7, i8, i9, i10, i11, i12, i13, i14, i15, i16, i17, i18, i19, i20, i21, i22, i23, i24, i25, i26, i27, i28, i29, i30, i31, i32\r\n\nRemote-control command(s):\nCALCulate:NRMMw:MEAS<i>:MEValuation:LIST:MODulation:EVM:DMRS:LOW:EXTReme?"}, {"Level"=5, "Class Only"=FALSE, "Identifier"="RSCMXPNRFR2M_ATTR_FETCH_MULTI_EVAL_MEASUREMENT_LIST_EVM_PEAK_HIGH_AVERAGE_RESULTS", "Descriptive Name"="Fetch Multi Eval Measurement List EVM Peak High Average Results", "Data Type"=enum."RawString", "Command"="FETC:NRMM:MEAS{instance}:MEV:LIST:MOD:EVM:PEAK:HIGH:AVER?", "Access"=enum."Read Only", "Range Table"="", "Read Callback"="", "Write Callback"="", "Range Callback"="", "Check Callback"="", "Rngtable Callback"="", "Coerce Callback"="", "Supported Models"="", "Instrument Options"="", "Check Status Callback"="", "Flags"=0, "Help"="Returns error vector magnitude peak values for low and high EVM window position, for all measured list mode segments.\n\nAvailable Repeated Capabilities:\ninstance: i0, i1, i2, i3, i4, i5, i6, i7, i8, i9, i10, i11, i12, i13, i14, i15, i16, i17, i18, i19, i20, i21, i22, i23, i24, i25, i26, i27, i28, i29, i30, i31, i32\r\n\nRemote-control command(s):\nFETCh:NRMMw:MEAS<i>:MEValuation:LIST:MODulation:EVM:PEAK:HIGH:AVERage?"}, {"Level"=5, "Class Only"=FALSE, "Identifier"="RSCMXPNRFR2M_ATTR_FETCH_MULTI_EVAL_MEASUREMENT_LIST_EVM_PEAK_HIGH_CURRENT_RESULTS", "Descriptive Name"="Fetch Multi Eval Measurement List EVM Peak High Current Results", "Data Type"=enum."RawString", "Command"="FETC:NRMM:MEAS{instance}:MEV:LIST:MOD:EVM:PEAK:HIGH:CURR?", "Access"=enum."Read Only", "Range Table"="", "Read Callback"="", "Write Callback"="", "Range Callback"="", "Check Callback"="", "Rngtable Callback"="", "Coerce Callback"="", "Supported Models"="", "Instrument Options"="", "Check Status Callback"="", "Flags"=0, "Help"="Returns error vector magnitude peak values for low and high EVM window position, for all measured list mode segments.\n\nAvailable Repeated Capabilities:\ninstance: i0, i1, i2, i3, i4, i5, i6, i7, i8, i9, i10, i11, i12, i13, i14, i15, i16, i17, i18, i19, i20, i21, i22, i23, i24, i25, i26, i27, i28, i29, i30, i31, i32\r\n\nRemote-control command(s):\nFETCh:NRMMw:MEAS<i>:MEValuation:LIST:MODulation:EVM:PEAK:HIGH:CURRent?"}, {"Level"=5,
